vi "Prepare Data for ParserSorter.vi"(7 "AE Groups to Include":i32[](array[numeric]), 8 "Error In":errorcluster, 11 "SRList":T6 {"SR#" format="%#_10g"}) -> (0 "Error Out":errorcluster, 3 "Prepared SR List":T1[](array[typedef]))   [LabVIEW 2017, in "Client.lvlib"]
uses:
  Client.lvlib
  ServerCommunications/TypeDefs/SR List.ctl
  ServerCommunications/TypeDefs/SR Data.ctl
  ParserSorter/SR Data.ctl
  ParserSorter/AE Group.ctl
  ParserSorter/SR Status.ctl
  ParserSorter/SR Level.ctl
  ParserSorter/SR Type.ctl
  ParserSorter/ParserSorter.lvlib
  ServerCommunications/CommsServer.lvlib
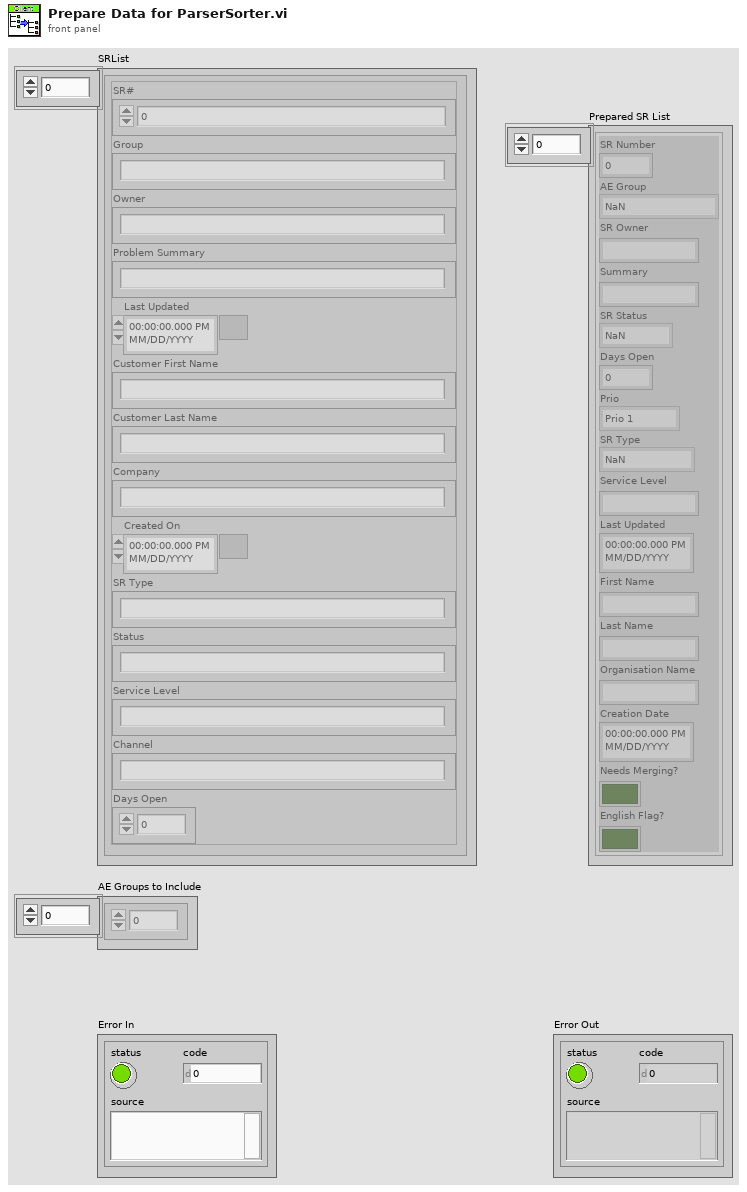
[diagram p1: front panel]
types:
  T1 = typedef "Client.lvlib/ParserSorter.lvlib/SR Data.ctl" = cluster{"SR Number":i64, "AE Group":T2, "SR Owner":string, "Summary":string, "SR Status":T3, "Days Open":dbl, "Prio":T4, "SR Type":T5, "Service Level":string, "Last Updated":timestamp, "First Name":string, "Last Name":string, "Organisation Name":string, "Creation Date":timestamp, "Needs Merging?":bool, "English Flag?":bool}
  T2 = typedef "Client.lvlib/ParserSorter.lvlib/AE Group.ctl" = enum32{"NaN", "AE-Germany", "AE-Poland", "AE-Switzerland", "AE-Czech Republic", "AE-Hungary", "AE-Romania", "AE-Slovakia", "AE-Slovenia"}
  T3 = typedef "Client.lvlib/ParserSorter.lvlib/SR Status.ctl" = enum32{"NaN", "Caller Abandoned", "Created in Error", "Declined to Purchase Support", "Expired", "Forum Resolved AE", "Forum Resolved Customer", "IN WORK", "IN WORK Collab with AES", "IN WORK Collab with PSE", "IN WORK Collab with SE", "IN WORK Escalation", "IN WORK Customer Added Note", "Open", "Potentially Resolved", "POC Resolved", "Resolved", "RMA Waiting on Customer", "RMA Open", "RMA In Progress", "RMA Closed - DOA", "RMA Closed", "RMA Approved for Return", "Project Complete", "Presumed Resolved", "IN WORK Wait on Customer"}
  T4 = typedef "Client.lvlib/ParserSorter.lvlib/SR Level.ctl" = enum16{"Prio 1", "Prio 2", "Prio 3", "Prio 4"}
  T5 = typedef "Client.lvlib/ParserSorter.lvlib/SR Type.ctl" = enum32{"NaN", "ATE Core Configurations (BYOATE)", "Activation", "BioBench", "CAN", "CM C Series", "Calibration", "Consulting Services", "CounterTimer", "DAQExpress", "DASYLab", "DIAdem", "DMM", "DSA HW", "Digital_IO", "FIRST (NIC Only)", "FieldBus", "FieldPoint", "Functional Savety", "GATI", "GPIB", "HMI and Industrial PCs", "HiQ", "HighSpeedDigital_IO", "IMAQ", "IOTech Vibration", "Industrial Communications", "InsightCM", "LV", "LV CD&Sim", "LV Comms", "LV Controls Add-Ons", "LV Embedded", "LV MathScript RT", "LV NXG", "LV NXT", "LVDSC", "LVFPGA", "LVPDA and LV Touch Panel", "LVRT", "LabWindows_CVI", "Lookout", "MATRIXx", "MStudioDotNet", "MStudioVisualBasic", "MStudioVisualC", "Measure (Legacy)", "Motion", "MultifunctionDAQ", "Multimedia Test HW/SW", "Multisim (EWB)", "NI Update Service", "OPC Servers", "Optical (OSI)", "PXI Controllers, Chassis, MXI", "PXI Timing and Sync", "Power Supplies and SMUs", "Powertrain Controls", "RAID", "RF", "RF Software", "RIO", "SC Express", "SCC", "SCXI", "SPEEDY-33 (Hyperception)", "STS", "ScopeDigitizers", "Serial", "Signal Sources", "SignalCondOther", "SignalExpress", "Software Defined Intruments", "Sound and Vibration SW", "Switch Executive", "Switches", "TestStand", "USRP", "Ultiboard (EWB)", "VBench", "VI Logger", "VXI_MXI", "VeriStand", "VisionSW", "VolumeLicenseMgr", "WSN", "Web UI Builder", "myRIO"}
  T6 = typedef "Client.lvlib/CommsServer.lvlib/SR List.ctl" = T7[]
  T7 = typedef "Client.lvlib/CommsServer.lvlib/SR Data.ctl" = cluster{"SR#":dbl, "Group":string, "Owner":string, "Problem Summary":string, "Last Updated":timestamp, "Customer First Name":string, "Customer Last Name":string, "Company":string, "Created On":timestamp, "SR Type":string, "Status":string, "Service Level":string, "Channel":string, "Days Open":dbl}
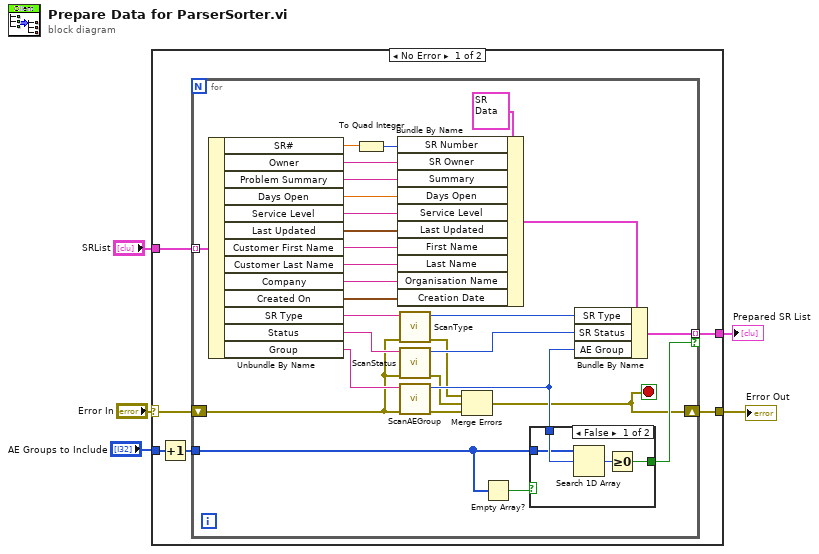
[diagram p0: block diagram]
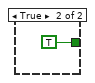
[diagram p2: hidden frame]
diagram:
  n1 = case shown="No Error" "Error In" {
    selector: "Error In" -> [w9 w46]
    tunnel: [w8 w46] -> w4
    tunnel: "SRList" -> [w11 _]
    tunnel: [w10 _] -> w2
    tunnel: "AE Groups to Include" -> [w7 _]
    frame No Error {
      n2 = Increment(x=w7) -> (x+1=w6:i32[])
      n3 = for {
        tunnel: w11 -> [w40] mode=indexing
        tunnel: [w24] -> w10 mode=indexing if=w23
        shift-right: [w14] -> w8
        shift-left: w9 -> [w16]
        tunnel: w6 -> [w22]
        stop <- w14 stop-if-true
        n4 = Unbundle By Name(w40) -> ("SR#"=w37:dbl, "Owner"=w35:string, "Problem Summary"=w34:string, "Days Open"=w33:dbl, "Service Level"=w32:string, "Last Updated"=w31:timestamp, "Customer First Name"=w30:string, "Customer Last Name"=w29:string, "Company"=w28:string, "Created On"=w27:timestamp, "SR Type"=w18:string, "Status"=w26:string, "Group"=w20:string)
        n5 = To Quad Integer(1:w37) -> (0:w36:i64)
        n6 = Bundle By Name(cluster=T1 {"SR Number"=0, "AE Group"=enum."NaN", "SR Owner"="", "Summary"="", "SR Status"=enum."Open", "Days Open"=0.0, "Prio"=enum."Prio 1", "SR Type"=enum."OPC Servers", "Service Level"="", "Last Updated"=timestamp(0 s since 1904-01-01), "First Name"="", "Last Name"="", "Organisation Name"="", "Creation Date"=timestamp(0 s since 1904-01-01), "Needs Merging?"=FALSE, "English Flag?"=FALSE} ("SR Number"), "SR Number"=w36, "SR Owner"=w35, "Summary"=w34, "Days Open"=w33, "Service Level"=w32, "Last Updated"=w31, "First Name"=w30, "Last Name"=w29, "Organisation Name"=w28, "Creation Date"=w27) -> (w38:T1)
        n7 = call "ScanType.vi"("error in (no error)"=w16, "Type String"=w18) -> ("error out"=w12:errorcluster, "SR Type"=w17:T5)  [unwired: 8 in]
        n8 = call "ScanStatus.vi"("error in (no error)"=w16, "Status String"=w26) -> ("error out"=w13:errorcluster, "SR Status"=w25:T3)  [unwired: 8 in]
        n9 = call "ScanAEGroup.vi"("error in (no error)"=w16, "AE Group String"=w20) -> ("error out"=w15:errorcluster, "AE Group"=w19:T2)  [unwired: 8 in]
        n10 = Merge Errors(w12, w13, w15) -> (w14:errorcluster)
        n11 = Empty Array?(array=w22) -> (empty?=w21:bool)
        n12 = case shown="False" w21 {
          tunnel: w19 -> [w44 _]
          tunnel: [w42 TRUE] -> w23
          tunnel: w22 -> [w41 _]
          frame False {
            n13 = Search 1D Array(1D array=w41, element=w44) -> (index of element=w43:i32)  [unwired: 1 in]
            n14 = Greater Or Equal To 0?(x=w43) -> (x >= 0?=w42:bool)
          }
          frame True {
          }
        }
        n15 = Bundle By Name(cluster=w38, "SR Type"=w17, "SR Status"=w25, "AE Group"=w19) -> (w24:T1)
      }
    }
    frame Error {
    }
  }
  "Error Out" <- w4
  "Prepared SR List" <- w2
